vi "Include Motor Physical Calc.vi"(10 "Motor Torque":dbl[unit], 11 "Physical Values":T1 {"Moment of Inertia (kg m^2)" format="%#_3p"}) -> (2 "Angular Accel":dbl[unit], 3 "Flywheel Torque":dbl[unit])   [LabVIEW 2020]
uses:
  Motor Physical Values.ctl
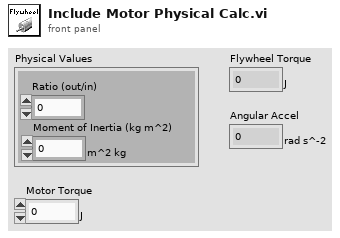
[diagram p1: front panel]
types:
  T1 = typedef "Motor Physical Values.ctl" = cluster{"Ratio (out/in)":dbl, "Moment of Inertia (kg m^2)":dbl[unit]}
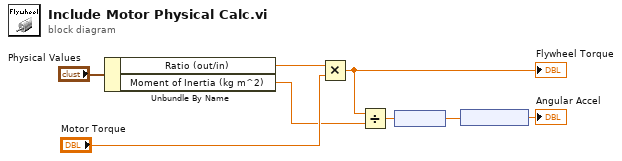
[diagram p0: block diagram]
diagram:
  n1 = Unbundle By Name("Physical Values") -> ("Ratio (out/in)"=w2:dbl, "Moment of Inertia (kg m^2)"=w3:dbl[unit])
  n2 = Multiply(x=w2, y="Motor Torque") -> (x*y=w5:dbl[unit])
  "Flywheel Torque" <- w5
  n3 = Divide(x=w5, y=w3) -> (x/y=w6:dbl[unit])
  n4 = node(w6) -> (w7:dbl)
  n5 = node(w7) -> (→"Angular Accel":dbl[unit])
